vi "DFD Integer Delay (Array NChan).vi"(7 "init? (F)":bool, 8 "error in (no error)":errorcluster, 10 "delay":i32, 11 "signal in":dbl[][](array[numeric])) -> (0 "error out":errorcluster, 3 "signal out":dbl[][](array[numeric]))   [LabVIEW 2017, in "NI_DigFilterLicensed.lvlib"]
doc: "Delays a signal continuously by a specified integer number of sample intervals. Wire data to the <B>signal in</B> input to determine the polymorphic instance to use or manually select the instance."
uses:
  <vilib>/addons/Digital Filter Design/NI_DigFilterLicensed.lvlib
  <vilib>/addons/Digital Filter Design/Process.llb/DFD Integer Delay with State (Array).vi
  <vilib>/addons/Digital Filter Design/NI_DigFilter_Process.lvlib
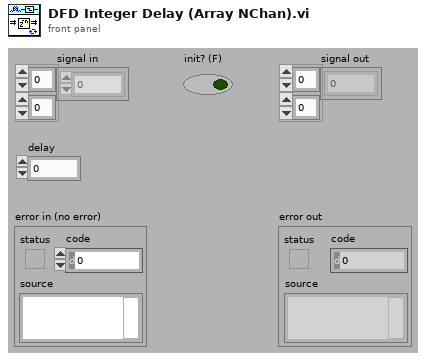
[diagram p1: front panel]
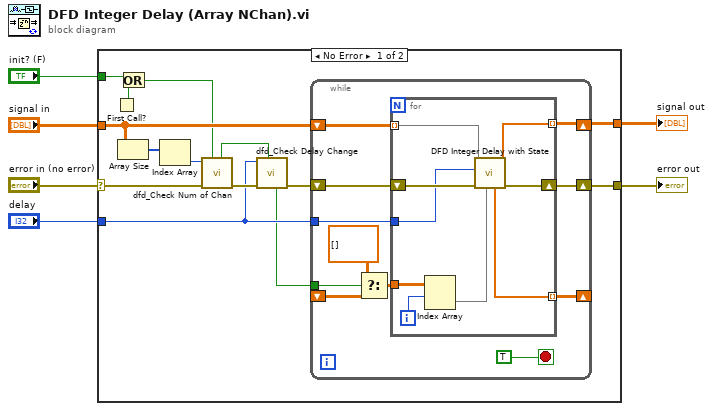
[diagram p0: block diagram]
diagram:
  n1 = case shown="No Error" "error in (no error)" {
    selector: "error in (no error)" -> [w12 w41]
    tunnel: [w20 w41] -> w5
    tunnel: "signal in" -> [w16 _]
    tunnel: [w19 _] -> w3
    tunnel: "delay" -> [w9 _]
    tunnel: "init? (F)" -> [w18 _]
    frame No Error {
      n2 = First Call?() -> (First Call?: T/F=w17:bool)
      n3 = Array Size(array=w16) -> (size(s)=w15:i32[])
      n4 = Or(x=w18, y=w17) -> (x .or. y?=w13:bool)
      n5 = Index Array(array=w15) -> (element=w14:i32)  [unwired: 1 in]
      n6 = call <vilib>:"dfd_Check Num of Chan.vi"("init in"=w13, "error in (no error)"=w12, "#ch in"=w14) -> ("error out"=w11:errorcluster, "init out"=w8:bool)  [unwired: 7 out]
      n7 = call <vilib>:"dfd_Check Delay Change.vi"("init in"=w8, "error in (no error)"=w11, "delay in"=w9) -> ("error out"=w10:errorcluster, "init out"=w7:bool)  [unwired: 7 out]
      n8 = while {
        shift-right: [w30] -> _
        shift-left: _ -> [w28]
        tunnel: w7 -> [w24]
        tunnel: w9 -> [w25]
        shift-right: [w26] -> w19
        shift-left: w16 -> [w23]
        shift-right: [w22] -> w20
        shift-left: w10 -> [w29]
        stop <- TRUE stop-if-true
        n9 = Select(t=dbl[][] [], s=w24, f=w28) -> (s? t:f=w27:dbl[][])
        n10 = for {
          tunnel: [w40] -> w30 mode=indexing
          tunnel: w27 -> [w37]
          tunnel: w23 -> [w32] mode=indexing
          tunnel: [w35] -> w26 mode=indexing
          tunnel: w25 -> [w34]
          shift-right: [w38] -> w22
          shift-left: w29 -> [w39]
          i -> [w33]
          n11 = Index Array(array=w37, index (row)=w33) -> (element=w36:dbl[])  [unwired: 1 in]
          n12 = call-poly <vilib>:"DFD Integer Delay with State.vi"("state in"=w36, "error in (no error)"=w39, "delay"=w34, "signal in"=w32) -> ("error out"=w38:errorcluster, "signal out"=w35:dbl[], "state out"=w40:dbl[])  [unwired: 5 out]
        }
      }
    }
    frame Error {
    }
  }
  "error out" <- w5
  "signal out" <- w3
